vi "Find Delta Samples of Rising Edge.vi"(10 "Channel 2":waveform(dbl), 11 "Channel 1":waveform(dbl)) -> (3 "Sample Offset":dbl)   [LabVIEW 2023]
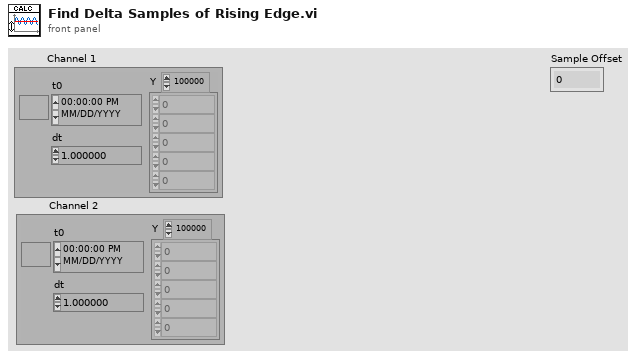
[diagram p1: front panel]
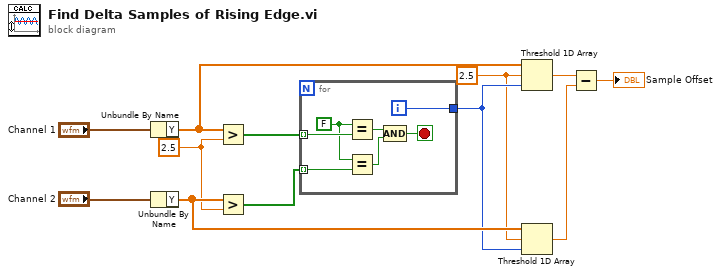
[diagram p0: block diagram]
diagram:
  w1 = 2.5 ("threshold y")
  w2 = 2.5
  n1 = Unbundle By Name("Channel 1") -> ("Y"=w10:dbl[])
  n2 = Unbundle By Name("Channel 2") -> ("Y"=w9:dbl[])
  n3 = Greater?(x=w10, y=w2) -> (0:w5:bool[])
  n4 = Greater?(x=w9, y=w2) -> (0:w4:bool[])
  n5 = for {
    tunnel: w5 -> [w19] mode=indexing
    tunnel: w4 -> [w18] mode=indexing
    tunnel: [w17] -> w3
    i -> [w17]
    stop <- w14 stop-if-true
    w13 = FALSE ("x")
    n6 = Equal?(x=w13, y=w19) -> (x = y?=w16:bool)
    n7 = Equal?(x=w13, y=w18) -> (x = y?=w15:bool)
    n8 = Compound Arithmetic op=AND(w16, w15) -> (w14:bool)
  }
  n9 = Threshold 1D Array(1:w3, 2:w1, 3:w10) -> (0:w8:dbl)
  n10 = Threshold 1D Array(1:w3, 2:w1, 3:w9) -> (0:w7:dbl)
  n11 = Subtract(x=w8, y=w7) -> (x-y=→"Sample Offset":dbl)
